vi "example_vector_search_vectors.vi"() -> ()   [LabVIEW 2020]
uses:
  src/vectorstore/abstract_vector_base/abstract_vector_base.lvclass
  src/models/llm_openai_embedding/llm_openai_embedding.lvclass
  D:/Personal/LabVIEW LLMs/src/models/abstract_llm_base/abstract_llm_base.lvclass
  src/vectorstore/vector_qdrant/vector_qdrant.lvclass
  D:/Personal/LabVIEW LLMs/src/vectorstore/abstract_vector_base/abstract_vector_base.lvclass
  src/models/message_text/message_text.lvclass
  D:/Personal/LabVIEW LLMs/src/models/abstract_message_base/abstract_message_base.lvclass
  src/models/message_vectors/message_vectors.lvclass
  src/models/llm_openai_embedding/Instantiate_llm_openai_embed.vi
  src/models/message_text/create_text_message.vi
  src/models/message_vectors/get_vector_message_value.vi
  src/utilities/env_variables/env_variables.lvlib
  src/models/abstract_llm_embedding/abstract_llm_embedding.lvclass
  D:/Personal/LabVIEW LLMs/src/models/message_vectors/message_vectors.lvclass
panel:
  in  "K size":u32=3
  out "Search Results":string[](array[string])
  in  "Search Query":string="Yellow Fruit"
  out "error out":errorcluster
  in  "collection_name":string="my_collection"
  in  "Vector Selector":enum32{"qdrant", "weviate"}(tab)
  in  "host_url":string="http://localhost:6333/"
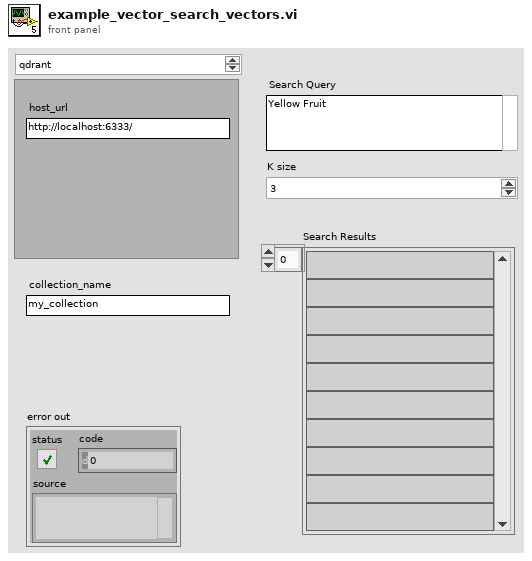
[diagram p1: front panel]
types:
  T1 = typedef "message_vectors.lvclass/embedding.ctl" = cluster{"index":u32, "Vectors":dbl[]}
  T2 = typedef "abstract_vector_base.lvclass/search result.ctl" = cluster{"score":dbl, "vector":T3}
  T3 = typedef "abstract_vector_base.lvclass/vector.ctl" = cluster{"id":string, "vector":dbl[], "text":string, "metadata":cluster{"key":string, "value":string}[]}
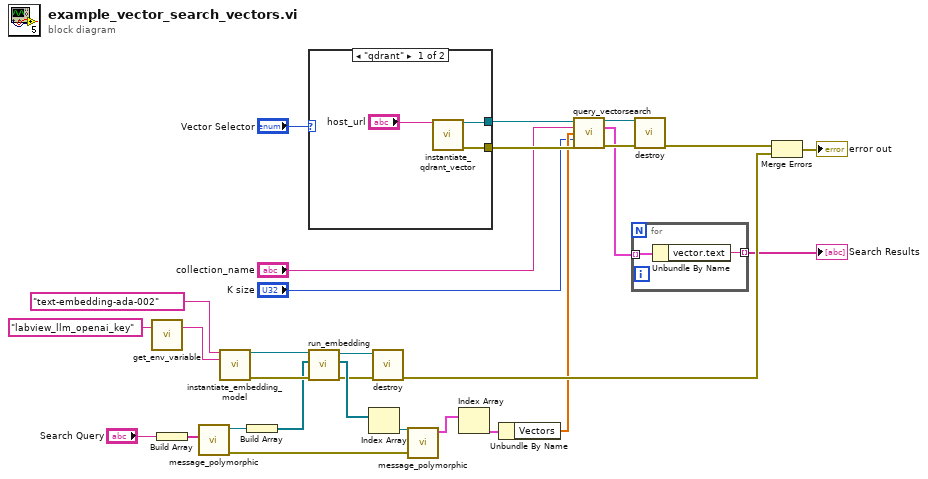
[diagram p0: block diagram]
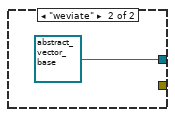
[diagram p2: hidden frame]
diagram:
  n1 = call "get_env_variable.vi"("Environment Variable Name"="labview_llm_openai_key") -> ("Value"=w22:string)  [unwired: 1 in, 1 out]
  n2 = Build Array("Search Query") -> (w15:string[])
  n3 = call-poly "message_polymorphic.vi"("content"=w15) -> ("error out"=w10:errorcluster, "message_text out"=w14:refnum<class "message_text.lvclass">)  [unwired: 9 in]
  n4 = call-poly "instantiate_embedding_model.vi"("model_name"="text-embedding-ada-002", "openai_key"=w22) -> ("llm_openai_embedding out"=w24:refnum<class "llm_openai_embedding.lvclass">, "error out"=w25:errorcluster)  [unwired: 12 in]
  n5 = Build Array(w14) -> (w13:refnum<class "message_text.lvclass">[])
  n6 = case shown="\"qdrant\"" "Vector Selector" {
    tunnel: [w32 refnum<class "abstract_vector_base.lvclass"> refnum ("abstract_vector_base.lvclass")] -> w27
    tunnel: [w30 _] -> w26
    frame "qdrant" {
      n7 = call "instantiate_qdrant_vector.vi"("host_url"="host_url") -> ("vector_qdrant out"=w32:refnum<class "vector_qdrant.lvclass">, "error out"=w30:errorcluster)  [unwired: 13 in]
    }
    frame "weviate" {
    }
  }
  n8 = call "run_embedding.vi"("error in (no error)"=w25, "Messages"=w13, "abstract_llm_embedding in"=w24) -> ("error out"=w5:errorcluster, "Response"=w12:refnum<class "message_vectors.lvclass">[], "abstract_llm_embedding out"=w4:refnum<class "llm_openai_embedding.lvclass">)  [unwired: 6 in]
  n9 = Index Array(array=w12) -> (element=w11:refnum<class "message_vectors.lvclass">)  [unwired: 1 in]
  n10 = call-dynamic "destroy.vi"("error in (no error)"=w5, "llm_openai_embedding in"=w4) -> ("error out"=w19:errorcluster)  [unwired: 8 in, 1 out]
  n11 = call-poly "message_polymorphic.vi"("error in (no error)"=w10, "message_vectors in"=w11) -> ("embedding_data"=w9:T1[])  [unwired: 8 in, 1 out]
  n12 = Index Array(array=w9) -> (element=w8:T1)  [unwired: 1 in]
  n13 = Unbundle By Name(w8) -> ("Vectors"=w7:dbl[])
  n14 = call-dynamic "query_vectorsearch.vi"("abstract_vector_base in"=w27, "collection_name"="collection_name", "vector"=w7, "limit"="K size", "error in (no error)"=w26) -> ("abstract_vector_base out"=w18:refnum<class "abstract_vector_base.lvclass">, "results"=w3:T2[], "error out"=w17:errorcluster)  [unwired: 8 in]
  n15 = for {
    tunnel: w3 -> [w35] mode=indexing
    tunnel: [w34] -> w2 mode=indexing
    n16 = Unbundle By Name(w35) -> ("vector.text"=w34:string)
  }
  "Search Results" <- w2
  n17 = call-dynamic "destroy.vi"("abstract_vector_base in"=w18, "error in (no error)"=w17) -> ("error out"=w28:errorcluster)  [unwired: 12 in, 1 out]
  n18 = Merge Errors(w28, w19) -> (→"error out":errorcluster)
